vi "set pulse from memory memory write.vi"(8 "error in (no error)":errorcluster, 11 "device_type in":refnum<class "device_type.lvclass">) -> (0 "error out":errorcluster, 2 "IQ data to memory":u64[](array[numeric]), 3 "device_type out":refnum<class "device_type.lvclass">)   [LabVIEW 2021, in "device_type.lvclass"]
uses:
  device_type.lvclass
  device_type.lvclass/device_type.ctl
  <vilib>/addons/Modulation/Analog/controls/Complex Data Waveform.ctl
  <instrlib>/_niInstr/DSP/v1/Shared/Public/IQ Data.ctl
  <vilib>/addons/Modulation/Analog/support/Validators/mod_Fractional Resample Validate.vi
  <vilib>/addons/Modulation/Analog/support/Validators/mod_Check Flush State.vi
  <vilib>/addons/Modulation/Analog/support/mod_FractionalResampler.vi
  <vilib>/addons/Modulation/Analog/support/mod_Integer Rate Interpolation.vi
  <vilib>/addons/Modulation/Analog/support/mod_Set Error Source.vi
  <vilib>/addons/Modulation/Analog/support/Validators/mod_Validate Complex Waveform.vi
  <vilib>/addons/Modulation/Analog/support/mod_PerformResampling.vi
  <vilib>/addons/Modulation/Analog/support/Validators/mod_WFErrorHandler.vi
  <vilib>/sound2/lvsound2.llb/Sound File Read Open.vi
  <vilib>/sound2/lvsound2.llb/Sound File Read (DBL).vi
  <vilib>/Utility/error.llb/Error Cluster From Error Code.vi
  <vilib>/addons/Modulation/Analog/support/mod_Resampling Factors.vi
  <vilib>/addons/Modulation/Analog/support/mod_ResamplingFilter.vi
  <vilib>/addons/Modulation/Analog/support/mod_Generate Integer Interpolation Filter.vi
  <instrlib>/_niInstr/DSP/v1/FPGA/Public/Sub VIs/Data Conversion/IQ to U32 - 1 spc - S18.1.vi
  <vilib>/addons/Modulation/niAMT.lvlib
  <instrlib>/_niInstr/DSP/v1/FPGA/niInstr DSP v1 FPGA.lvlib
  <instrlib>/_niInstr/DSP/v1/Shared/niInstr DSP v1 Shared.lvlib
panel:
  out "Waveform Graph":cluster{"t0":dbl, "dt":dbl, "Y":dbl[]}[](graph)
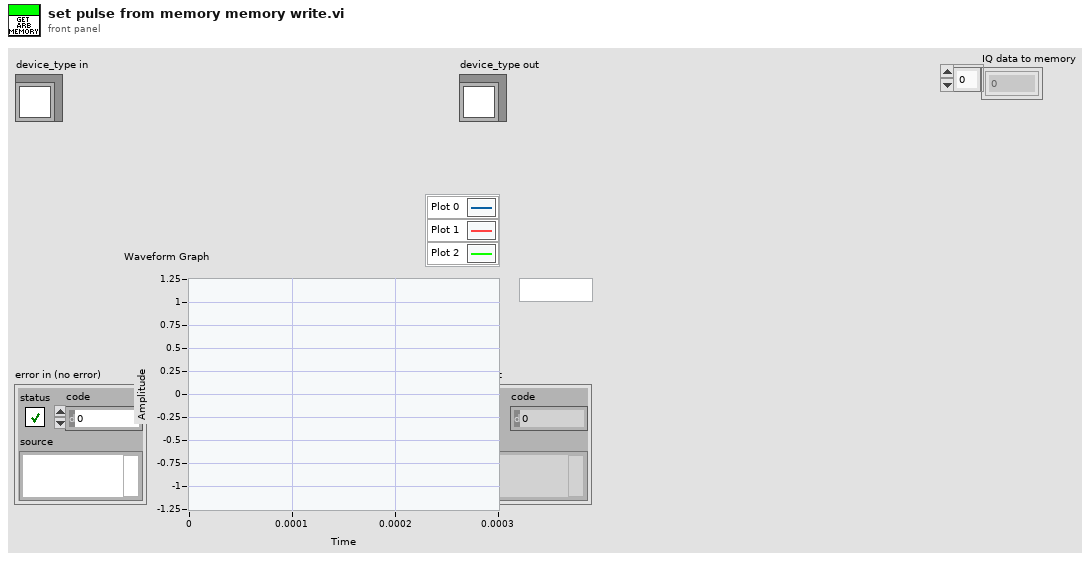
[diagram p1: front panel]
types:
  T1 = typedef "niAMT.lvlib/Complex Data Waveform.ctl" = cluster{"t0":dbl, "dt":dbl, "Y":cdb[]}
  T2 = typedef "niInstr DSP v1 Shared.lvlib/IQ Data.ctl" = cluster{"I":fxp<+/-,18,1>, "Q":fxp<+/-,18,1>, "overflow":bool}
  T3 = typedef "Sound File Refnum.ctl" = refnum<file>
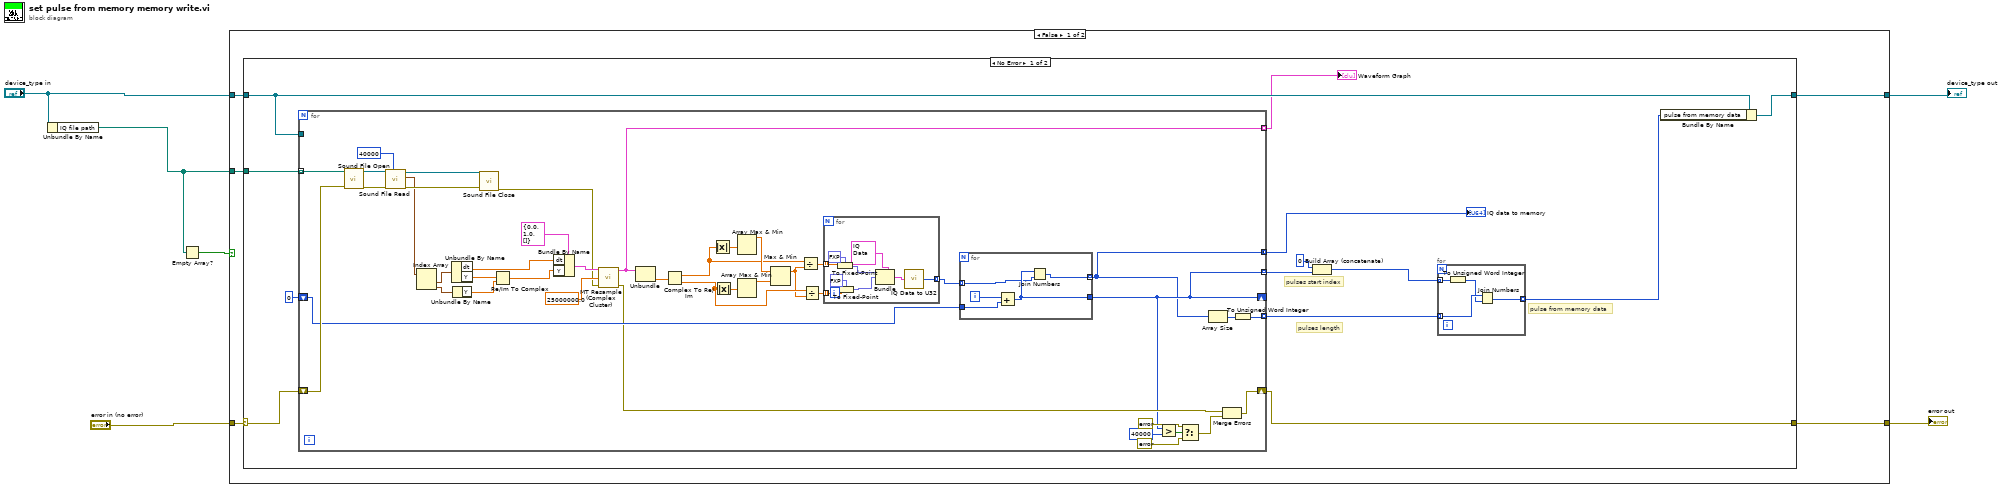
[diagram p0: block diagram]
diagram:
  n1 = Unbundle By Name("device_type in") -> ("IQ file path"=w3:path[])
  n2 = Empty Array?(array=w3) -> (empty?=w5:bool)
  n3 = case shown="False" w5 {
    tunnel: "error in (no error)" -> [w11 w87]
    tunnel: "device_type in" -> [w10 w88]
    tunnel: w3 -> [w9 _]
    tunnel: [w8 w88] -> w2
    tunnel: [w7 w87] -> w1
    frame False {
      n4 = case shown="No Error" w11 {
        selector: w11 -> [w24 w86]
        tunnel: [w21 w86] -> w7
        tunnel: [w16 w85] -> w8
        tunnel: w10 -> [w18 w85]
        tunnel: w9 -> [w13 _]
        frame No Error {
          # "pulse from memory data"
          # "pulses start index"
          # "pulses length"
          n5 = for {
            shift-right: [w37] -> w21
            shift-left: w24 -> [w62]
            tunnel: w13 -> [w46] mode=indexing
            shift-right: [w36] -> _
            shift-left: 0 -> [w44]
            tunnel: [w36] -> w23 mode=indexing
            tunnel: w18 -> [_]
            tunnel: [w35] -> w12 mode=concatenating
            tunnel: [w29] -> w19 mode=indexing
            tunnel: [w34] -> w14 mode=indexing
            n6 = call-poly <vilib>:"Sound File Open.vi"("error in (no error)"=w62, "path"=w46) -> ("error out"=w67:errorcluster, "sound file refnum"=w70:T3)  [unwired: 8 in]
            n7 = call-poly <vilib>:"Sound File Read.vi"("number of samples/ch (-1: all)"=40000, "error in (no error)"=w67, "sound file refnum"=w70) -> ("error out"=w66:errorcluster, "data"=w65:waveform(dbl)[], "sound file refnum out"=w69:T3)  [unwired: 4 in, 2 out]
            n8 = Index Array(array=w65) -> (element #1=w64:waveform(dbl), element #2=w63:waveform(dbl))  [unwired: 2 in]
            n9 = Unbundle By Name(w64) -> ("dt"=w58:dbl, "Y"=w61:dbl[])
            n10 = Unbundle By Name(w63) -> ("Y"=w60:dbl[])
            n11 = call <vilib>:"Sound File Close.vi"("error in (no error)"=w66, "sound file refnum"=w69) -> ("error out"=w47:errorcluster)  [unwired: 9 in]
            n12 = Re/Im To Complex(1:w60, 2:w61) -> (0:w57:cdb[])
            n13 = Bundle By Name(cluster=T1 {"t0"=0.0, "dt"=1.0, "Y"=[]} ("input complex waveform"), "dt"=w58, "Y"=w57) -> (w56:T1)
            n14 = call <vilib>:"MT Resample (Complex Cluster).vi"("input complex waveform"=w56, "desired sample rate (Hz)"=25000000.0, "error in (no error)"=w47) -> ("output complex waveform"=w34:T1, "error out"=w38:errorcluster)  [unwired: 11 in]
            n15 = Unbundle(w34) -> ("Y"=w54:cdb[])  [unwired: 2 out]
            n16 = Complex To Re/Im(x + iy=w54) -> (x=w49:dbl[], y=w48:dbl[])
            n17 = Absolute Value(x=w49) -> (abs(x)=w51:dbl[])
            n18 = Absolute Value(x=w48) -> (abs(x)=w50:dbl[])
            n19 = Array Max & Min(array=w51) -> (max value=w52:dbl)  [unwired: 3 out]
            n20 = Array Max & Min(array=w50) -> (max value=w53:dbl)  [unwired: 3 out]
            n21 = Max & Min(x=w52, y=w53) -> (max(x,y)=w45:dbl)  [unwired: 1 out]
            n22 = Divide(x=w49, y=w45) -> (x/y=w32:dbl[])
            n23 = Divide(x=w48, y=w45) -> (x/y=w33:dbl[])
            n24 = for {
              tunnel: w33 -> [w77] mode=indexing
              tunnel: w32 -> [w74] mode=indexing
              tunnel: [w71] -> w31 mode=indexing
              n25 = To Fixed-Point(fixed-point type=fxp<+/-,18,1> 0.0 ("I"), number=w74) -> (fixed-point=w73:fxp<+/-,18,1>)
              n26 = To Fixed-Point(fixed-point type=fxp<+/-,18,1> 0.0 ("I"), number=w77) -> (fixed-point=w78:fxp<+/-,18,1>)
              n27 = Bundle(cluster=T2 {"I"=0.0, "Q"=0.0, "overflow"=FALSE} ("IQ data"), "I"=w73, "Q"=w78) -> (w72:T2)  [unwired: 1 in]
              n28 = call-poly <instrlib>:"IQ Data to U32.vi"("IQ data"=w72) -> ("U32 data"=w71:u32)  [unwired: 13 in, 1 out]
            }
            n29 = for {
              tunnel: [w84] -> w35 mode=indexing
              tunnel: [w82] -> w36
              tunnel: w44 -> [w81]
              tunnel: w31 -> [w80] mode=indexing
              i -> [w83]
              n30 = Add(x=w83, y=w81) -> (x+y=w82:i32)
              n31 = Join Numbers(hi=w82, lo=w80) -> ((hi.lo)=w84:u64)
            }
            n32 = Greater?(x=w36, y=40000) -> (0:w42:bool)
            n33 = Select(t=errorcluster {"status"=FALSE, "code"=5052, "source"="too meny sampels"}, s=w42, f=errorcluster {"status"=FALSE, "code"=0, "source"=""} ("error out")) -> (s? t:f=w39:errorcluster)
            n34 = Array Size(array=w35) -> (size(s)=w30:i32)
            n35 = Merge Errors(w38, w39) -> (w37:errorcluster)
            n36 = To Unsigned Word Integer(number=w30) -> (unsigned 16bit integer=w29:u16)
          }
          "Waveform Graph" <- w14
          "IQ data to memory" <- w12
          n37 = Build Array (concatenate)(0, w23) -> (w20:i32[])
          n38 = for {
            tunnel: w20 -> [w26] mode=indexing
            tunnel: w19 -> [w28] mode=indexing
            tunnel: [w27] -> w17 mode=indexing
            n39 = To Unsigned Word Integer(number=w26) -> (unsigned 16bit integer=w25:u16)
            n40 = Join Numbers(hi=w28, lo=w25) -> ((hi.lo)=w27:u32)
          }
          n41 = Bundle By Name(cluster=w18, "pulse from memory data"=w17) -> (w16:refnum<class "device_type.lvclass">)
        }
        frame Error {
        }
      }
    }
    frame True {
    }
  }
  "device_type out" <- w2
  "error out" <- w1
